vi "FilterChannelsByDataGroup.vi"(8 "error in (no error)":errorcluster, 10 "group":string, 11 "device model":T4) -> (0 "error out":errorcluster, 3 "channels in data group":T1[](array[typedef]))   [LabVIEW 2017, in "DeviceModelHelpers.lvlib"]
doc: "Returns properties for the channels that belong to a specific data group, including channels that belong to multiple data groups."
uses:
  <vilib>/addons/InsightCM/Utilities/DeviceModelHelpers/DeviceModelHelpers.lvlib
  <vilib>/addons/InsightCM/MessageBus/Base/controls/R2_DeviceModel.ctl
  <vilib>/addons/InsightCM/MessageBus/Base/controls/R2_Device.ctl
  <vilib>/addons/InsightCM/MessageBus/Base/controls/KeyValuePair.ctl
  <vilib>/addons/InsightCM/MessageBus/Base/controls/DeviceState.ctl
  <vilib>/addons/InsightCM/MessageBus/Base/controls/R2_DataGroup.ctl
  <vilib>/addons/InsightCM/MessageBus/Base/controls/OperatingState.ctl
  <vilib>/addons/InsightCM/MessageBus/Base/controls/Trigger.ctl
  <vilib>/addons/InsightCM/MessageBus/Base/controls/Condition.ctl
  <vilib>/addons/InsightCM/MessageBus/Base/controls/BurstModeTrigger.ctl
  <vilib>/addons/InsightCM/MessageBus/Base/controls/R2_Channel.ctl
  <vilib>/addons/InsightCM/MessageBus/Base/controls/Metric.ctl
  <vilib>/addons/InsightCM/MessageBus/Base/controls/Tag.ctl
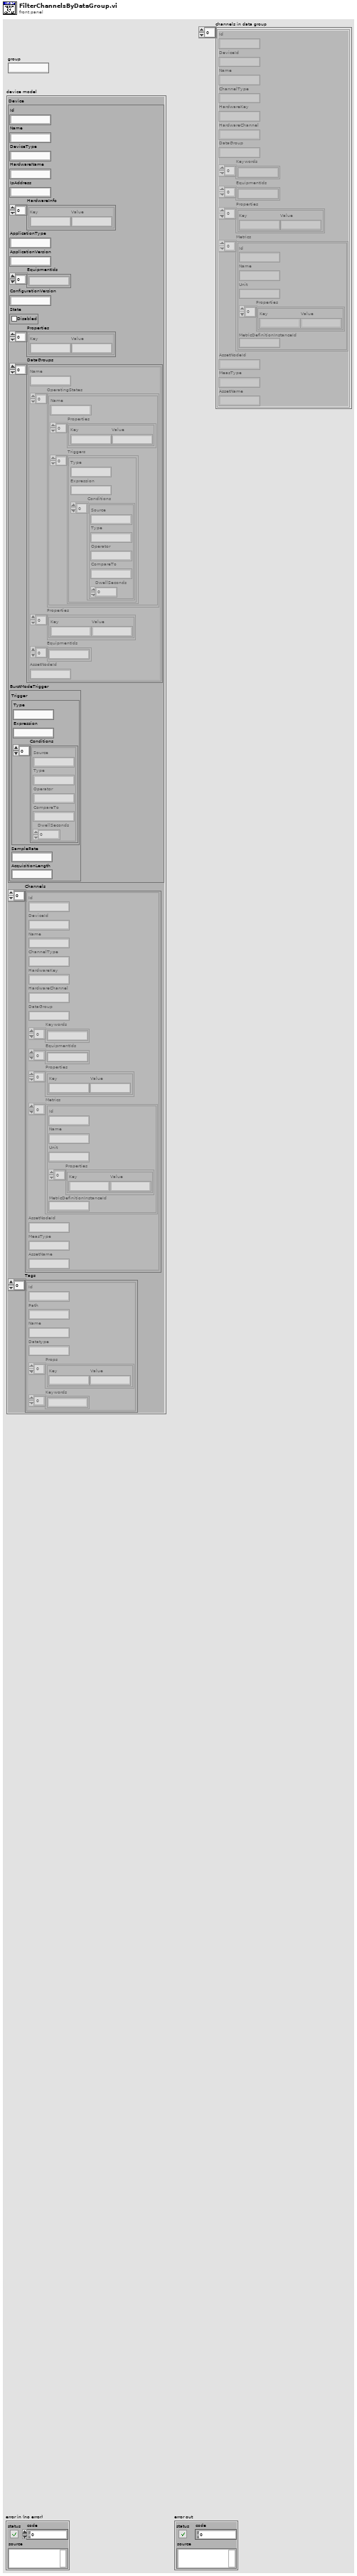
[diagram p1: front panel]
types:
  T1 = typedef "R2_Channel.ctl" = cluster{"Id":string, "DeviceId":string, "Name":string, "ChannelType":string, "HardwareKey":string, "HardwareChannel":string, "DataGroup":string, "Keywords":string[], "EquipmentIds":string[], "Properties":T2[], "Metrics":T3[], "AssetNodeId":string, "MeasType":string, "AssetName":string}
  T2 = typedef "KeyValuePair.ctl" = cluster{"Key":string, "Value":string}
  T3 = typedef "Metric.ctl" = cluster{"Id":string, "Name":string, "Unit":string, "Properties":T2[], "MetricDefinitionInstanceId":string}
  T4 = typedef "R2_DeviceModel.ctl" = cluster{"Device":T5, "Channels":T1[], "Tags":T12[]}
  T5 = typedef "R2_Device.ctl" = cluster{"Id":string, "Name":string, "DeviceType":string, "HardwareName":string, "IpAddress":string, "HardwareInfo":T2[], "ApplicationType":string, "ApplicationVersion":string, "EquipmentIds":string[], "ConfigurationVersion":string, "State":T6, "Properties":T2[], "DataGroups":T7[], "BurstModeTrigger":T11}
  T6 = typedef "DeviceState.ctl" = cluster{"Disabled":bool}
  T7 = typedef "R2_DataGroup.ctl" = cluster{"Name":string, "OperatingStates":T8[], "Properties":T2[], "EquipmentIds":string[], "AssetNodeId":string}
  T8 = typedef "OperatingState.ctl" = cluster{"Name":string, "Properties":T2[], "Triggers":T9[]}
  T9 = typedef "Trigger.ctl" = cluster{"Type":string, "Expression":string, "Conditions":T10[]}
  T10 = typedef "Condition.ctl" = cluster{"Source":string, "Type":string, "Operator":string, "CompareTo":string, "DwellSeconds":dbl}
  T11 = typedef "BurstModeTrigger.ctl" = cluster{"Trigger":T9, "SampleRate":string, "AcquisitionLength":string}
  T12 = typedef "Tag.ctl" = cluster{"Id":string, "Path":string, "Name":string, "Datatype":string, "Props":T2[], "Keywords":string[]}
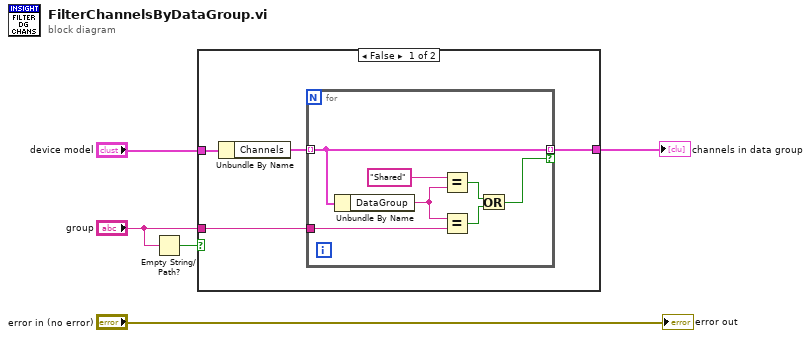
[diagram p0: block diagram]
diagram:
  n1 = Empty String/Path?(string/path="group") -> (empty?=w2:bool)
  n2 = case shown="False" w2 {
    tunnel: "device model" -> [w9 _]
    tunnel: "group" -> [w7 _]
    tunnel: [w6 _] -> w1
    frame False {
      n3 = Unbundle By Name(w9) -> ("Channels"=w8:T1[])
      n4 = for {
        tunnel: w8 -> [w15] mode=indexing
        tunnel: w7 -> [w16]
        tunnel: [w15] -> w6 mode=indexing if=w10
        n5 = Unbundle By Name(w15) -> ("DataGroup"=w14:string)
        n6 = Equal?(x="Shared", y=w14) -> (x = y?=w12:bool)
        n7 = Equal?(x=w14, y=w16) -> (x = y?=w11:bool)
        n8 = Or(x=w12, y=w11) -> (x .or. y?=w10:bool)
      }
    }
    frame True {
    }
  }
  "channels in data group" <- w1
  "error out" <- "error in (no error)"
